vi "Rawdata_Generator_2.vi"() -> ()   [LabVIEW 2020]
uses:
  ctl/Image_Configuration.ctl
  ctl/Image_EBD_Config.ctl
panel:
  out "Index":i32
  in  "Lines of Post-EBD Data":u16
  in  "Lines of Pre-EBD Data":u16
  in  "Base Imagedata Binary File":path
  in  "Post EBD File":path
  in  "Pre EBD File":path
  in  "stop":bool
  out "Progress":dbl(slide) scale=0.0..100.0
  out "error out":errorcluster
  in  "Output File Path":path
  in  "Timestamp Type":enum16{"Base", "Base +/- Rand(Delta T)"}(ring)
  in  "Delta T (ns)":u64=1000000
  in  "Base Relative Time (ns)":u64=33333333
  in  "Num of Frames to generate":u32=5000
  in  "T0":timestamp=timestamp(3761222400 s since 1904-01-01)
  in  "Image Data Type":u8=44 format="%x"
  in  "Image Configuration":T1={"Width"=1920, "Height"=1536}
  # "30 FPS\n33.333333 ms"
  # "1 ms"
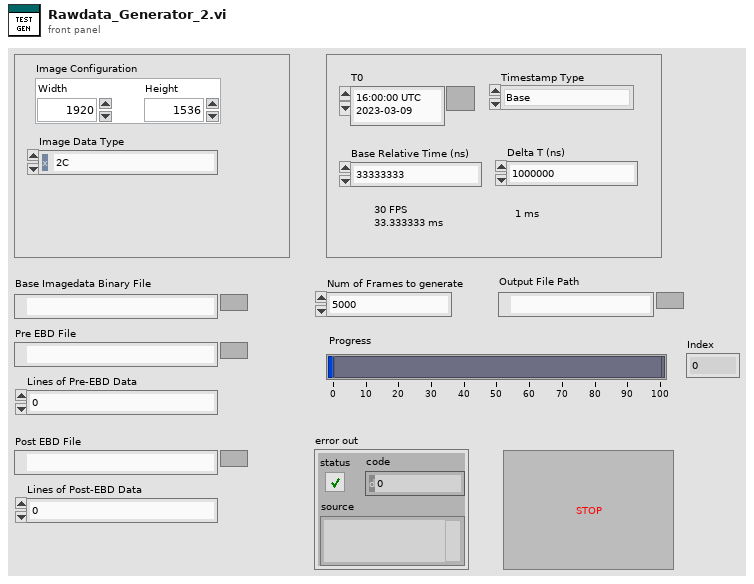
[diagram p1: front panel]
types:
  T1 = typedef "Image_Configuration.ctl" = cluster{"Width":i32, "Height":i32}
  T2 = typedef "Image_EBD_Config.ctl" = cluster{"Lines of Pre-EBD Data":u16, "Lines of Post-EBD Data":u16, "Total EBD Block Size":u32, "Pre-EBD Block Offset ":u32, "Post-EBD Block Offset ":u32}
  T3 = enum16{"open", "replace", "create", "open or create", "replace or create", "replace or create with confirmation"}
  T4 = enum16{"big-endian, network order", "native, host order", "little-endian"}
  T5 = typedef "Image_Data_Config.ctl" = cluster{"Lines of Image Data":u16, "Bytes per Even Line":u16, "Bytes per Odd Line":u16, "Image Data Type":u8, "Total Image Data Block Size":u32, "Image Data Block Offset":u32}
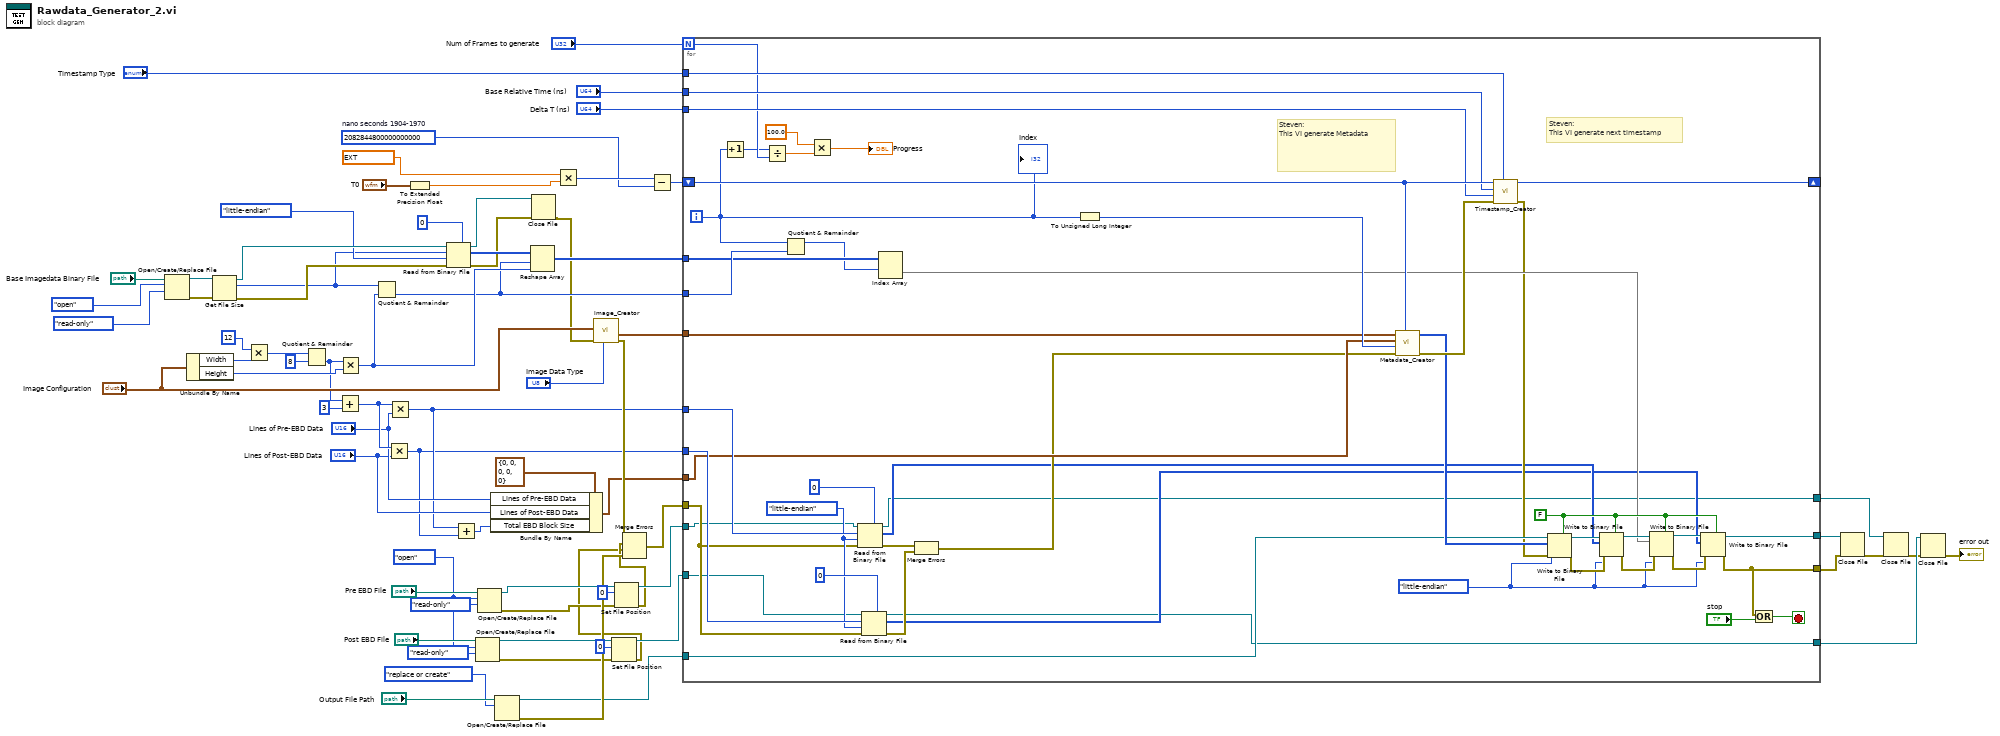
[diagram p0: block diagram]
diagram:
  w34 = T3."open" ("operation (0:open)")
  w69 = u64 2082844800000000000  # nano seconds 1904-1970
  n1 = Open/Create/Replace File(file path (use dialog)="Base Imagedata Binary File", operation (0:open)=T3."open", access (0:read/write)=enum16{"read/write", "read-only", "write-only"}."read-only") -> (refnum out=w59:refnum<file>, error out=w60:errorcluster)  [unwired: 3 in, 1 out]
  n2 = Unbundle By Name("Image Configuration") -> ("Width"=w58:i32, "Height"=w54:i32)
  n3 = Get File Size(file=w59, error in=w60) -> (refnum out=w52:refnum<file>, size (in bytes)=w49:i64, 0:w51:errorcluster)
  n4 = Multiply(x=12, y=w58) -> (x*y=w56:i32)
  n5 = Quotient & Remainder(x=w56, y=8) -> (floor(x/y)=w31:i32)  [unwired: 1 out]
  n6 = Add(x=w31, y=3) -> (x+y=w29:i32)
  n7 = Multiply(x=w31, y=w54) -> (x*y=w46:i32)
  n8 = Quotient & Remainder(x=w49, y=w46) -> (floor(x/y)=w42:i64)  [unwired: 1 out]
  n9 = Multiply(x=w29, y="Lines of Post-EBD Data") -> (x*y=w23:i32)
  n10 = Multiply(x=w29, y="Lines of Pre-EBD Data") -> (x*y=w24:i32)
  n11 = To Extended Precision Float(1:"T0") -> (0:w70:ext)
  n12 = Read from Binary File(5:u8 0, 8:w51, 9:T4."little-endian" ("byte order (0:big-endian, network order)"), 10:w49, 11:w52) -> (0:w38:errorcluster, 2:w47:u8[], 3:w39:refnum<file>)  [unwired: 1 in, 1 out]
  n13 = Add(x=w24, y=w23) -> (x+y=w22:i32)
  n14 = Open/Create/Replace File(file path (use dialog)="Post EBD File", operation (0:open)=w34, access (0:read/write)=enum16{"read/write", "read-only", "write-only"}."read-only") -> (refnum out=w7:refnum<file>, error out=w6:errorcluster)  [unwired: 3 in, 1 out]
  n15 = Open/Create/Replace File(file path (use dialog)="Pre EBD File", operation (0:open)=w34, access (0:read/write)=enum16{"read/write", "read-only", "write-only"}."read-only") -> (refnum out=w12:refnum<file>, error out=w11:errorcluster)  [unwired: 3 in, 1 out]
  n16 = Bundle By Name(cluster=T2 {"Lines of Pre-EBD Data"=0, "Lines of Post-EBD Data"=0, "Total EBD Block Size"=0, "Pre-EBD Block Offset "=0, "Post-EBD Block Offset "=0} ("EBD Config"), "Lines of Pre-EBD Data"="Lines of Pre-EBD Data", "Lines of Post-EBD Data"="Lines of Post-EBD Data", "Total EBD Block Size"=w22) -> (w21:T2)
  n17 = Open/Create/Replace File(file path (use dialog)="Output File Path", operation (0:open)=T3."replace or create") -> (refnum out=w28:refnum<file>, error out=w32:errorcluster)  [unwired: 4 in, 1 out]
  n18 = Reshape Array(w47, w42, w46) -> (w45:u8[][])
  n19 = Close File(refnum=w39, error in=w38) -> (error out=w37:errorcluster)  [unwired: 1 out]
  n20 = Multiply(x=ext 1000000000.0, y=w70) -> (x*y=w71:u64)
  n21 = call "Image_Creator.vi"("Image Data Type"="Image Data Type", "error in (no error)"=w37, "Image Configuration"="Image Configuration") -> ("error out"=w33:errorcluster, "Image Data Config"=w53:T5)  [unwired: 5 in, 2 out]
  n22 = Set File Position(offset (in bytes) (0)=i64 0, refnum=w7, error in=w6) -> (refnum out=w4:refnum<file>, error out=w3:errorcluster)  [unwired: 1 in]
  n23 = Set File Position(offset (in bytes) (0)=i64 0, refnum=w12, error in=w11) -> (refnum out=w9:refnum<file>, error out=w8:errorcluster)  [unwired: 1 in]
  n24 = Merge Errors(w33, w8, w3, w32) -> (w20:errorcluster)
  n25 = Subtract(x=w71, y=w69) -> (x-y=w66:u64)
  n26 = for {
    N: "Num of Frames to generate" -> [w107]
    shift-right: [w116] -> _
    shift-left: w66 -> [w120]
    tunnel: "Timestamp Type" -> [w119]
    tunnel: "Base Relative Time (ns)" -> [w118]
    tunnel: "Delta T (ns)" -> [w117]
    tunnel: [w102] -> w18
    tunnel: w53 -> [w99]
    tunnel: w45 -> [w97]
    tunnel: w42 -> [w98]
    tunnel: w24 -> [w92]
    tunnel: w23 -> [w89]
    tunnel: w9 -> [w75]
    tunnel: w4 -> [w74]
    tunnel: w28 -> [w82]
    tunnel: w21 -> [w87]
    tunnel: w20 -> [w86]
    tunnel: [w78] -> w19
    tunnel: [w77] -> w16
    tunnel: [w76] -> w15
    i -> [w96]
    stop <- w101 stop-if-true
    w88 = T4."little-endian" ("byte order (0:big-endian, network order)")
    w109 = FALSE ("prepend array or string size? (T)")
    w108 = T4."little-endian" ("byte order (0:big-endian, network order)")
    # "Steven:\nThis VI generate Metadata"
    # "Steven:\nThis VI generate next timestamp"
    n27 = Increment(x=w96) -> (x+1=w100:i32)
    n28 = Divide(x=w100, y=w107) -> (x/y=w106:dbl)
    n29 = Quotient & Remainder(x=w96, y=w98) -> (x-y*floor(x/y)=w95:i64)  [unwired: 1 out]
    n30 = Multiply(x=100.0, y=w106) -> (x*y=→"Progress":dbl)
    n31 = Read from Binary File(5:u8 0, 8:w86, 9:w88, 10:w92, 11:w75) -> (0:w85:errorcluster, 2:w80:u8[], 3:w77:refnum<file>)  [unwired: 1 in, 1 out]
    n32 = Read from Binary File(5:u8 0, 8:w86, 9:w88, 10:w89, 11:w74) -> (0:w84:errorcluster, 2:w79:u8[], 3:w76:refnum<file>)  [unwired: 1 in, 1 out]
    n33 = Index Array(array=w97, index (row)=w95) -> (element=w93:u8[])  [unwired: 1 in]
    n34 = Merge Errors(w85, w84) -> (w83:errorcluster)
    n35 = To Unsigned Long Integer(number=w96) -> (unsigned 32bit integer=w122:u32)
    n36 = call "Metadata_Creator.vi"("Frame Timestamp"=w120, "error in (no error)"=w83, "Frame Index"=w122, "EBD Config"=w87, "Image Data Config"=w99) -> ("error out"=w121:errorcluster, "Meta Data (U8)"=w94:u8[])  [unwired: 5 in]
    n37 = call "Timestamp_Creator.vi"("Timestamp Type"=w119, "error in (no error)"=w121, "Delta T (ns)"=w117, "Base Relative Time (ns)"=w118, "Previous Time (ns)"=w120) -> ("error out"=w81:errorcluster, "Next Time (ns)"=w116:u64)  [unwired: 5 in]
    n38 = Write to Binary File(file (use dialog)=w82, data=w94, error in=w81, 5:w109, 9:w108) -> (refnum out=w115:refnum<file>, error out=w114:errorcluster)  [unwired: 1 in, 1 out]
    n39 = Write to Binary File(file (use dialog)=w115, data=w80, error in=w114, 5:w109, 9:w108) -> (refnum out=w113:refnum<file>, error out=w112:errorcluster)  [unwired: 1 in, 1 out]
    n40 = Write to Binary File(file (use dialog)=w113, data=w93, error in=w112, 5:w109, 9:w108) -> (refnum out=w111:refnum<file>, error out=w110:errorcluster)  [unwired: 1 in, 1 out]
    n41 = Write to Binary File(file (use dialog)=w111, data=w79, error in=w110, 5:w109, 9:w108) -> (refnum out=w78:refnum<file>, error out=w102:errorcluster)  [unwired: 1 in, 1 out]
    n42 = Or(x=w102, y="stop") -> (x .or. y?=w101:bool)
    "Index" <- w96
  }
  n43 = Close File(refnum=w19, error in=w18) -> (error out=w17:errorcluster)  [unwired: 1 out]
  n44 = Close File(refnum=w16, error in=w17) -> (error out=w14:errorcluster)  [unwired: 1 out]
  n45 = Close File(refnum=w15, error in=w14) -> (error out=→"error out":errorcluster)  [unwired: 1 out]
